vi "New buffers NIringData.vi"(10 "data rate (hz)":dbl format="%#_13g", 11 "buffer (minutes)":dbl format="%#_13g") -> (2 "period (ms)":i32, 3 "ChannelMap":map{string, refnum<data-value>}(c390))   [LabVIEW 2021, in "RocketPlotDemo.lvlib"]
uses:
  RocketPlotDemo.lvlib
  <vilib>/National Instruments/Variant Ring Buffer/Ring Buffer.lvclass
  Demo Names.ctl
  ring buffer data.ctl
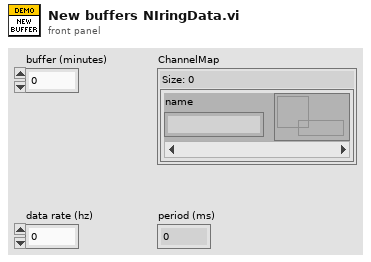
[diagram p1: front panel]
types:
  T1 = typedef "RocketPlotDemo.lvlib/Demo Names.ctl" = enum16{"Sine Wave", "Triangle Wave", "Sawtooth Wave", "Square Wave", "Uniform Noise", "Periodic Noise", "White Noise"}
  T2 = typedef "RocketPlotDemo.lvlib/ring buffer data.ctl" = cluster{"timestamp":dbl, "value":dbl}
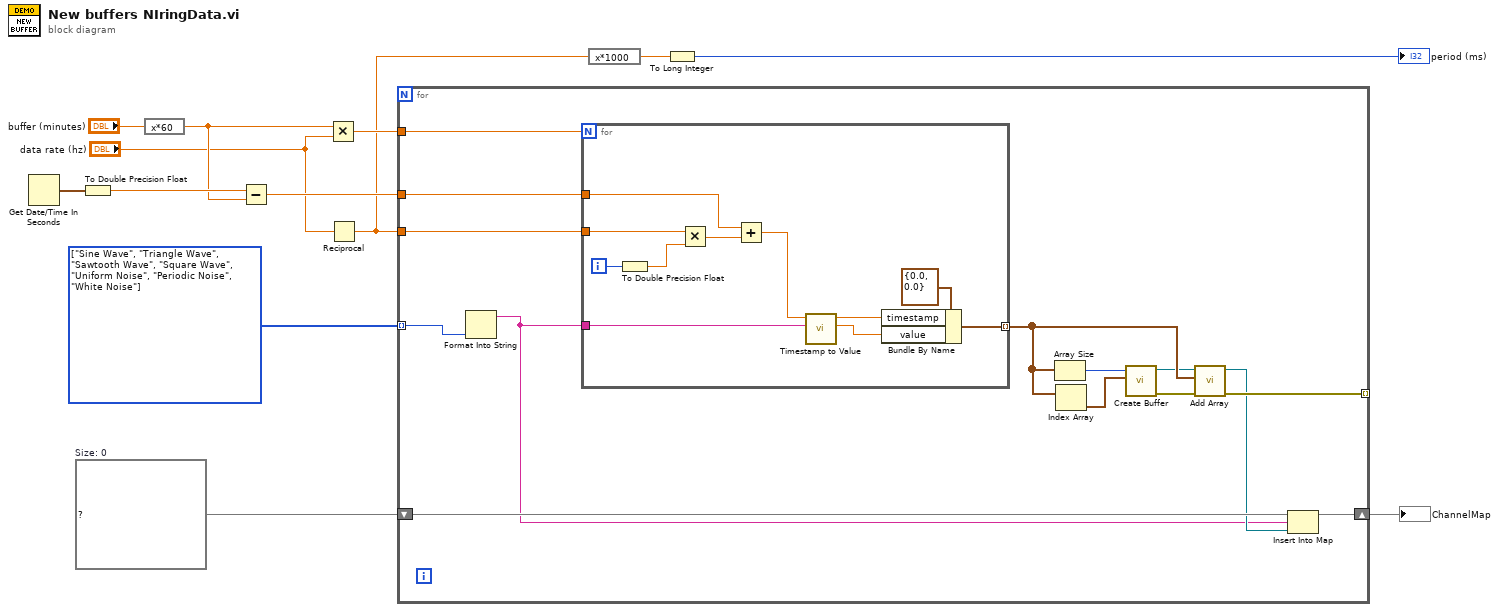
[diagram p0: block diagram]
diagram:
  w2 = map{string, refnum<data-value>} {}  # Size: 0
  w6 = T1[] [enum."Sine Wave", enum."Triangle Wave", enum."Sawtooth Wave", enum."Square Wave", enum."Uniform Noise", enum."Periodic Noise", enum."White Noise"] items=["Sine Wave", "Triangle Wave", "Sawtooth Wave", "Square Wave", "Uniform Noise", "Periodic Noise", "White Noise"]
  n1 = Get Date/Time In Seconds() -> (seconds since 1Jan1904=w13:timestamp)
  n2 = To Double Precision Float(number=w13) -> (double precision float=w11:dbl)
  n3 = expression code="x*60"("buffer (minutes)") -> (w10:dbl)
  n4 = Subtract(x=w11, y=w10) -> (x-y=w8:dbl)
  n5 = Multiply(x=w10, y="data rate (hz)") -> (x*y=w9:dbl)
  n6 = Reciprocal(x="data rate (hz)") -> (1/x=w5:dbl)
  n7 = for {
    tunnel: w9 -> [w27]
    tunnel: w8 -> [w18]
    tunnel: w5 -> [w26]
    tunnel: w6 -> [w15] mode=indexing
    tunnel: [w22] -> _ mode=indexing
    shift-right: [w20] -> w1
    shift-left: w2 -> [w21]
    n8 = Format Into String(w15) -> (resulting string=w14:string)  [unwired: 3 in, 1 out]
    n9 = for {
      N: w27 -> [_]
      tunnel: w26 -> [w38]
      tunnel: [w32] -> w24 mode=indexing
      tunnel: w18 -> [w30]
      tunnel: w14 -> [w28]
      i -> [w37]
      n10 = To Double Precision Float(number=w37) -> (double precision float=w36:dbl)
      n11 = Multiply(x=w38, y=w36) -> (x*y=w35:dbl)
      n12 = Add(x=w30, y=w35) -> (x+y=w29:dbl)
      n13 = call "Timestamp to Value.vi"("name"=w28, "timestamp"=w29) -> ("value"=w33:dbl, "timestamp (dup)"=w31:dbl)  [unwired: 8 in]
      n14 = Bundle By Name(cluster=T2 {"timestamp"=0.0, "value"=0.0} ("Cluster"), "timestamp"=w31, "value"=w33) -> (w32:T2)
    }
    n15 = Array Size(array=w24) -> (size(s)=w23:i32)
    n16 = Index Array(array=w24) -> (element=w25:T2)  [unwired: 1 in]
    n17 = call <vilib>:"Create Buffer.vi"("Data Type"=w25, "Buffer Size"=w23) -> ("Error In"=w16:errorcluster, "Ring Buffer Reference"=w17:refnum<data-value>)  [unwired: 8 in]
    n18 = call <vilib>:"Add Array.vi"("Error In"=w16, "Variants Array"=w24, "Ring Buffer Reference"=w17) -> ("Error Out"=w22:errorcluster, "Ring Buffer Reference"=w19:refnum<data-value>)  [unwired: 7 in]
    n19 = Insert Into Map(map in=w21, key=w14, value=w19) -> (map out=w20:map{string, refnum<data-value>})  [unwired: 2 out]
  }
  "ChannelMap" <- w1
  n20 = expression code="x*1000"(w5) -> (w4:dbl)
  n21 = To Long Integer(number=w4) -> (32bit integer=→"period (ms)":i32)
